vi "LabViewProject.vi"() -> ()   [LabVIEW 2024]
uses:
  <vilib>/Utility/error.llb/Trim Whitespace One-Sided.vi
  <vilib>/Instr/_visa.llb/VISA Configure Serial Port (Instr).vi
  <vilib>/Utility/file.llb/Read Delimited Spreadsheet (string).vi
  <vilib>/Utility/file.llb/Write Delimited Spreadsheet (string).vi
panel:
  in  "RFID_log_file_path":path
  out "concatenated string":string
  out "Boolean":bool
  out "serialCom":string
  in  "Voeg nieuwe kaart toe":bool
  out "all rows":string[][](array[string])
  in  "approved_RFID_file_path":path
  in  "stop":bool
  in  "Port":refnum<visa-resource-name>
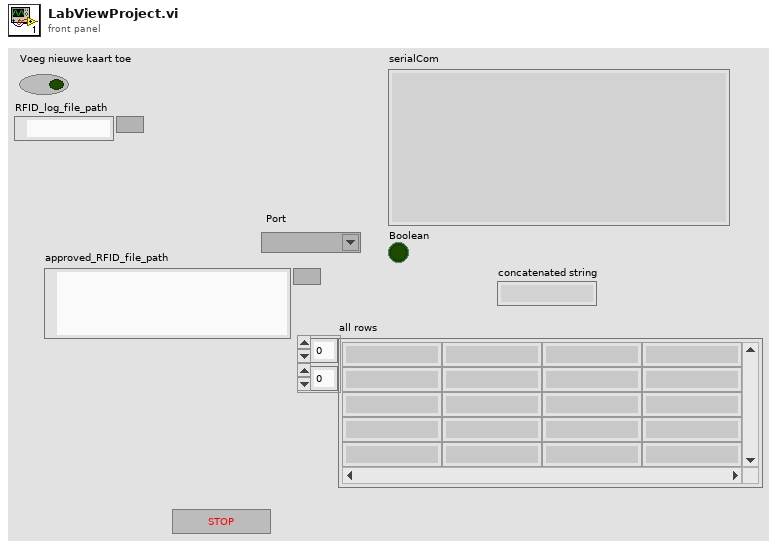
[diagram p1: front panel]
types:
  T1 = enum16{"initialize", "update_array", "checking_rfid", "access_granted", "add_new_rfid"}
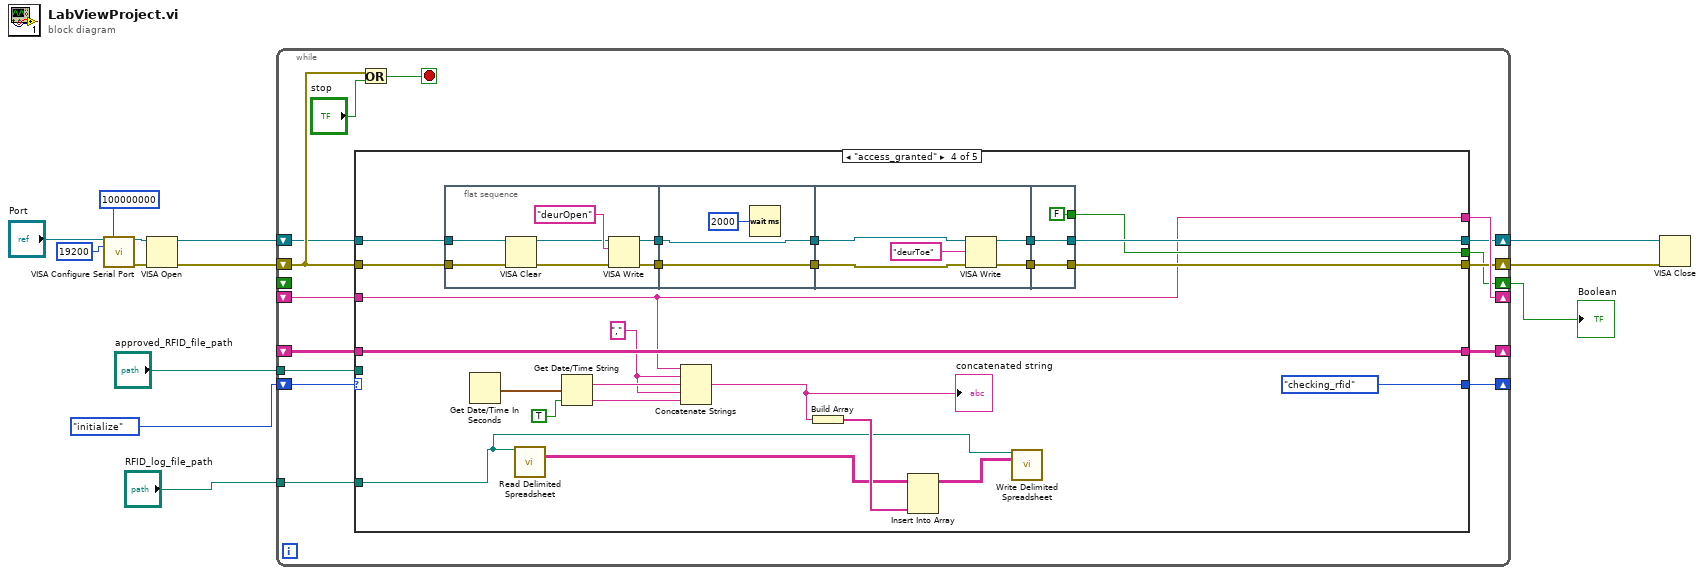
[diagram p0: block diagram]
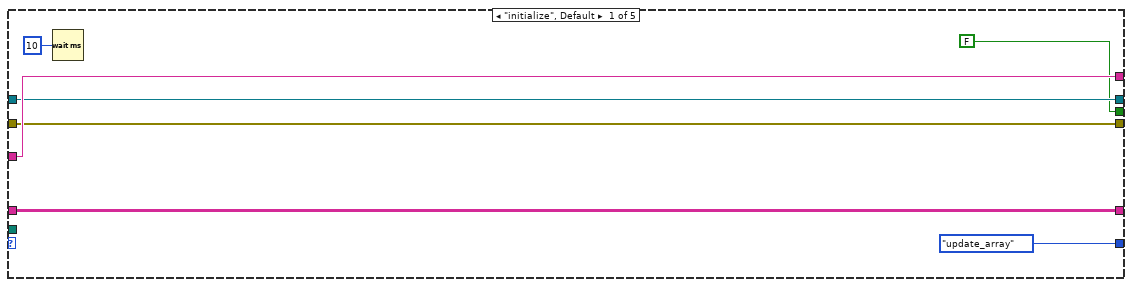
[diagram p2: hidden frame]
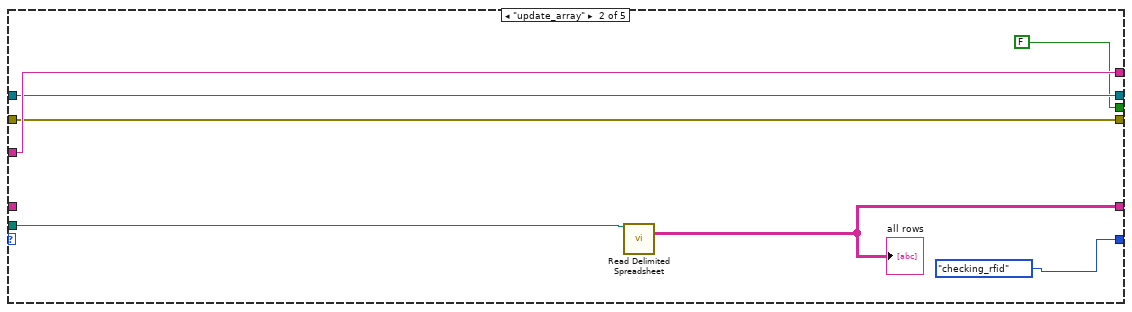
[diagram p3: hidden frame]
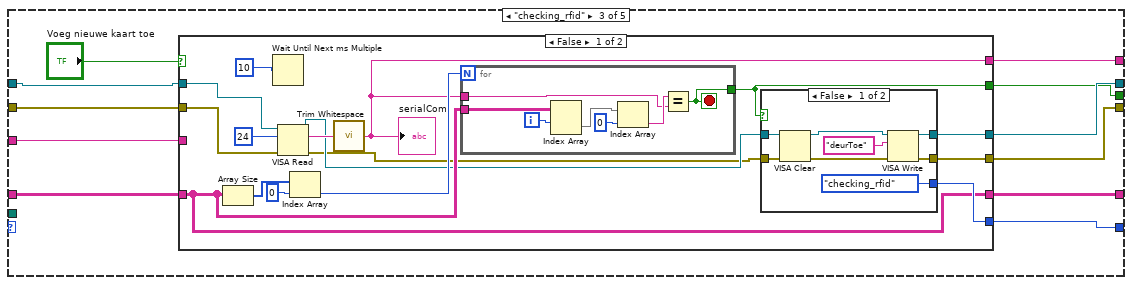
[diagram p4: hidden frame]
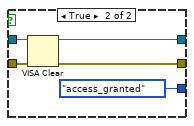
[diagram p5: hidden frame]
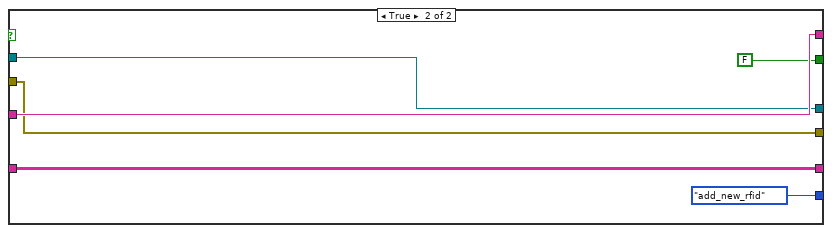
[diagram p6: hidden frame]
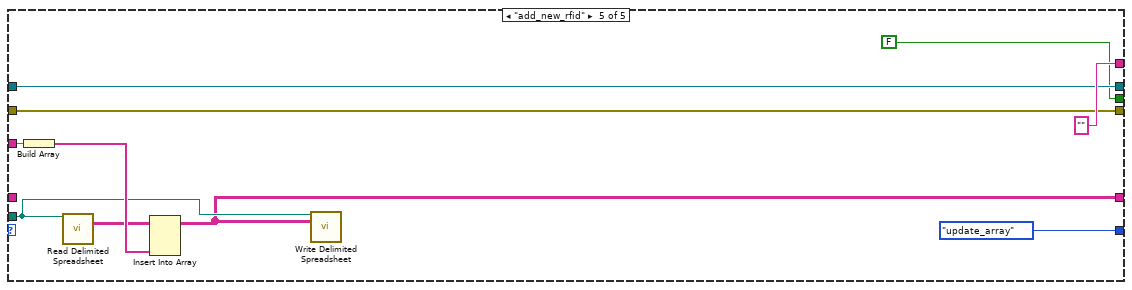
[diagram p7: hidden frame]
diagram:
  n1 = call-poly "VISA Configure Serial Port"("VISA resource name"="Port", "timeout (10sec)"=u32 100000000, "baud rate (9600)"=u32 19200) -> ("VISA resource name out"=w10:refnum<visa-resource-name>, "error out"=w9:errorcluster)  [unwired: 11 in]
  n2 = VISA Open(error in (no error)=w9, VISA resource name=w10) -> (VISA resource name=w12:refnum<visa-resource-name>, error out=w11:errorcluster)  [unwired: 3 in]
  n3 = while {
    tunnel: "approved_RFID_file_path" -> [w24]
    shift-right: [w25] -> _
    shift-left: T1."initialize" -> [w26]
    shift-right: [w19] -> _
    shift-left: _ -> [w23]
    shift-right: [w21] -> _
    shift-left: _ -> [w20]
    shift-right: [w17] -> w2
    shift-left: w12 -> [w18]
    shift-right: [w16] -> w3
    shift-left: w11 -> [w22]
    shift-right: [w15] -> w5
    shift-left: _ -> [_]
    tunnel: "RFID_log_file_path" -> [w14]
    stop <- w28 stop-if-true
    n4 = case shown="\"access_granted\"" w26 {
      tunnel: [T1."update_array" T1."checking_rfid" w48 T1."checking_rfid" T1."update_array"] -> w25
      tunnel: w24 -> [_ w42 _ _ w145]
      tunnel: w23 -> [w32 _ w51 w116 _]
      tunnel: w22 -> [w30 w37 w49 w119 w139]
      tunnel: w18 -> [w31 w38 w50 w118 w140]
      tunnel: [w33 w40 w52 w102 "" ("trimmed string")] -> w21
      tunnel: w20 -> [w33 w40 w47 w102 w143]
      tunnel: [w32 w39 w46 w116 w141] -> w19
      tunnel: [w31 w38 w45 w111 w140] -> w17
      tunnel: [w30 w37 w44 w110 w139] -> w16
      tunnel: [FALSE FALSE w43 w107 FALSE] -> w15
      tunnel: w14 -> [_ _ _ w97 _]
      frame "initialize", Default {
        n5 = Wait (ms)(milliseconds to wait=u32 10 ("millisecond multiple")) -> ()  [unwired: 1 out]
      }
      frame "update_array" {
        n6 = call-poly <vilib>:"Read Delimited Spreadsheet.vi"("file path (dialog if empty)"=w42) -> ("all rows"=w39:string[][])  [unwired: 9 in, 5 out]
        "all rows" <- w39
      }
      frame "checking_rfid" {
        n7 = case shown="False" "Voeg nieuwe kaart toe" {
          tunnel: [w54 w94] -> w52
          tunnel: w51 -> [w61 w93]
          tunnel: w50 -> [w64 w92]
          tunnel: w49 -> [w63 w91]
          tunnel: [w62 T1."add_new_rfid"] -> w48
          tunnel: w47 -> [_ w94]
          tunnel: [w61 w93] -> w46
          tunnel: [w58 w92] -> w45
          tunnel: [w57 w91] -> w44
          tunnel: [w56 FALSE] -> w43
          frame False {
            n8 = Array Size(array=w61) -> (size(s)=w68:i32[])
            n9 = Wait Until Next ms Multiple(millisecond multiple=u32 10) -> ()  [unwired: 1 out]
            n10 = VISA Read(VISA resource name=w64, byte count=u32 24, error in (no error)=w63) -> (VISA resource name out=w60:refnum<visa-resource-name>, read buffer=w66:string, error out=w59:errorcluster)  [unwired: 1 out]
            n11 = Index Array(array=w68, index=0) -> (element=w69:i32)
            n12 = call <vilib>:"Trim Whitespace.vi"("string"=w66) -> ("trimmed string"=w54:string)  [unwired: 1 in]
            "serialCom" <- w54
            n13 = for {
              N: w69 -> [_]
              tunnel: w54 -> [w83]
              tunnel: w61 -> [w89]
              tunnel: [w84] -> w56
              i -> [w85]
              stop <- w84 stop-if-true
              n14 = Index Array(array=w89, index (row)=w85) -> (element=w86:string[])  [unwired: 1 in]
              n15 = Index Array(array=w86, index=0) -> (element=w88:string)
              n16 = Equal?(x=w88, y=w83) -> (x = y?=w84:bool)
            }
            n17 = case shown="False" w56 {
              tunnel: [T1."checking_rfid" T1."access_granted"] -> w62
              tunnel: w60 -> [w76 w81]
              tunnel: w59 -> [w75 w80]
              tunnel: [w71 w79] -> w58
              tunnel: [w70 w78] -> w57
              frame False {
                n18 = VISA Clear(VISA resource name=w76, error in (no error)=w75) -> (VISA resource name out=w74:refnum<visa-resource-name>, error out=w73:errorcluster)
                n19 = VISA Write(VISA resource name=w74, write buffer="deurToe", error in (no error)=w73) -> (VISA resource name out=w71:refnum<visa-resource-name>, error out=w70:errorcluster)  [unwired: 1 out]
              }
              frame True {
                n20 = VISA Clear(VISA resource name=w81, error in (no error)=w80) -> (VISA resource name out=w79:refnum<visa-resource-name>, error out=w78:errorcluster)
              }
            }
          }
          frame True {
          }
        }
      }
      frame "access_granted" {
        w100 = "," ("string")
        n21 = flat-sequence {
          tunnel: w119 -> [w125]
          tunnel: w118 -> [w124]
          tunnel: [w121] -> w115
          tunnel: [w120] -> w112
          tunnel: w115 -> [w128]
          tunnel: [w128] -> w114
          tunnel: [w127] -> w113
          tunnel: w112 -> [w127]
          tunnel: w114 -> [w133]
          tunnel: w113 -> [w132]
          tunnel: [w131] -> w109
          tunnel: [w130] -> w108
          tunnel: [w136] -> w110
          tunnel: [w137] -> w111
          tunnel: w109 -> [w137]
          tunnel: w108 -> [w136]
          tunnel: [FALSE] -> w107
          frame #0 {
            n22 = VISA Clear(VISA resource name=w124, error in (no error)=w125) -> (VISA resource name out=w123:refnum<visa-resource-name>, error out=w122:errorcluster)
            n23 = VISA Write(VISA resource name=w123, write buffer="deurOpen", error in (no error)=w122) -> (VISA resource name out=w121:refnum<visa-resource-name>, error out=w120:errorcluster)  [unwired: 1 out]
          }
          frame #1 {
            n24 = Wait (ms)(milliseconds to wait=u32 2000) -> ()  [unwired: 1 out]
          }
          frame #2 {
            n25 = VISA Write(VISA resource name=w133, write buffer="deurToe", error in (no error)=w132) -> (VISA resource name out=w131:refnum<visa-resource-name>, error out=w130:errorcluster)  [unwired: 1 out]
          }
          frame #3 {
          }
        }
        n26 = Get Date/Time In Seconds() -> (seconds since 1Jan1904=w106:timestamp)
        n27 = call-poly <vilib>:"Read Delimited Spreadsheet.vi"("file path (dialog if empty)"=w97) -> ("all rows"=w103:string[][])  [unwired: 9 in, 5 out]
        n28 = Get Date/Time String(seconds (now)=w106, want seconds? (F)=TRUE) -> (date string=w101:string, time string=w99:string)  [unwired: 1 in]
        n29 = Concatenate Strings(w102, w100, w101, w100, w99) -> (w98:string)
        "concatenated string" <- w98
        n30 = Build Array(w98) -> (w104:string[])
        n31 = Insert Into Array(array=w103, new element=w104) -> (w96:string[][])  [unwired: 2 in]
        n32 = call-poly <vilib>:"Write Delimited Spreadsheet.vi"("file path (dialog if empty)"=w97, "2D data"=w96) -> ()  [unwired: 12 in, 2 out]
      }
      frame "add_new_rfid" {
        n33 = Build Array(w143) -> (w147:string[])
        n34 = call-poly <vilib>:"Read Delimited Spreadsheet.vi"("file path (dialog if empty)"=w145) -> ("all rows"=w146:string[][])  [unwired: 9 in, 5 out]
        n35 = Insert Into Array(array=w146, new element=w147) -> (w141:string[][])  [unwired: 2 in]
        n36 = call-poly <vilib>:"Write Delimited Spreadsheet.vi"("file path (dialog if empty)"=w145, "2D data"=w141) -> ()  [unwired: 12 in, 2 out]
      }
    }
    n37 = Or(x=w22, y="stop") -> (x .or. y?=w28:bool)
  }
  "Boolean" <- w5
  n38 = VISA Close(VISA resource name=w2, error in (no error)=w3) -> ()  [unwired: 1 out]
